vi "DisplayErrorsForMasterSlaveyes.vi"(0 "CmdLib In":refnum<k24>, 5 "Status:":refnum<vi>, 11 "error in":errorcluster) -> (4 "CmdLib Out":refnum<k24>, 15 "error out":errorcluster)   [LabVIEW 2021]
uses:
  C:/Program Files/New Focus/New Focus Picomotor Application/Samples/LabVIEW/Model 8742/LabVIEW 2009/CmdLib.dll
  Global Variablesyes.vi
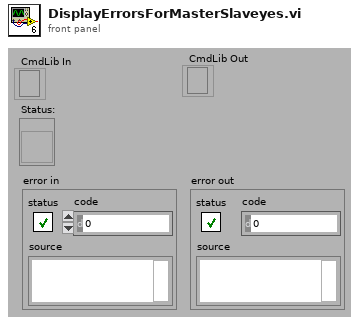
[diagram p1: front panel]
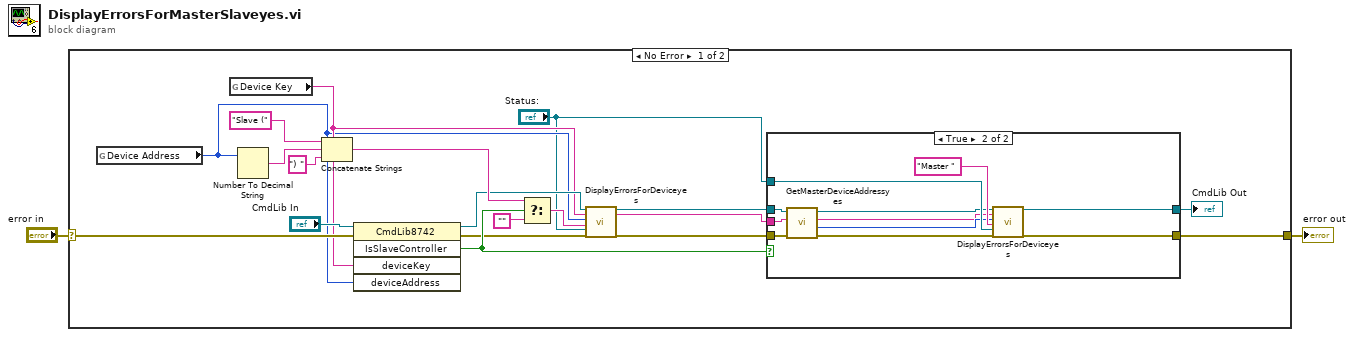
[diagram p0: block diagram]
diagram:
  n1 = case shown="No Error" "error in" {
    selector: "error in" -> [w20 w35]
    tunnel: [w4 w35] -> w2
    frame No Error {
      n2 = global read "Global Variablesyes.vi" "Device Address"() -> (w11:i32)
      n3 = global read "Global Variablesyes.vi" "Device Key"() -> (w12:string)
      n4 = Number To Decimal String(number=w11) -> (decimal integer string=w16:string)  [unwired: 1 in]
      n5 = Concatenate Strings("Slave (", w16, ") ") -> (w15:string)
      n6 = invoke class="CmdLib8742" method="IsSlaveController"(reference="CmdLib In", error in=w20, "deviceKey"=w12, "deviceAddress"=w11) -> (reference out=w13:refnum<k24>, error out=w10:errorcluster, "IsSlaveController"=w14:bool)  [unwired: 1 in, 2 out]
      n7 = Select(t=w15, s=w14, f="") -> (s? t:f=w9:string)
      n8 = call "DisplayErrorsForDeviceyes.vi"("CmdLib In"=w13, "Device Key"=w12, "Device Address"=w11, "Prefix"=w9, "Status:"="Status:", "error in"=w10) -> ("CmdLib Out"=w8:refnum<k24>, "DeviceKey Out"=w7:string, "error out"=w6:errorcluster)  [unwired: 10 in, 1 out]
      n9 = case shown="True" w14 {
        tunnel: w8 -> [w22 w29]
        tunnel: w7 -> [_ w28]
        tunnel: w6 -> [w23 w31]
        tunnel: "Status:" -> [_ w34]
        tunnel: [w23 w25] -> w4
        tunnel: [w22 w24] -> w3
        frame False {
        }
        frame True {
          n10 = call "GetMasterDeviceAddressyes.vi"("error in (no error)"=w31, "DeviceKey In"=w28, "CmdLib In"=w29) -> ("error out"=w30:errorcluster, "Device Address"=w32:i32, "DeviceKey Out"=w26:string, "CmdLib Out"=w27:refnum<k24>)  [unwired: 1 in]
          n11 = call "DisplayErrorsForDeviceyes.vi"("CmdLib In"=w27, "Device Key"=w26, "Device Address"=w32, "Prefix"="Master ", "Status:"=w34, "error in"=w30) -> ("CmdLib Out"=w24:refnum<k24>, "error out"=w25:errorcluster)  [unwired: 10 in, 2 out]
        }
      }
      "CmdLib Out" <- w3
    }
    frame Error {
    }
  }
  "error out" <- w2
